vi "BIO_new.vi"(8 "error in (no error)":errorcluster, 10 "*BIO_method":u64, 11 "SSL-Lib in":refnum<class "SSL-Lib.lvclass">) -> (0 "error out":errorcluster, 2 "BIO out":refnum<class "BIO.lvclass">, 3 "SSL-Lib out":refnum<class "SSL-Lib.lvclass">)   [LabVIEW 2013, in "SSL_Lib.lvlib" / "SSL-Lib.lvclass"]
uses:
  SSL-Lib.lvclass
  BIO/BIO.lvclass
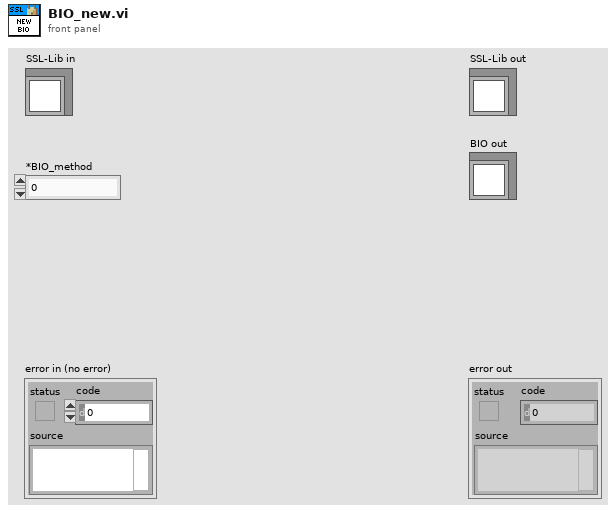
[diagram p1: front panel]
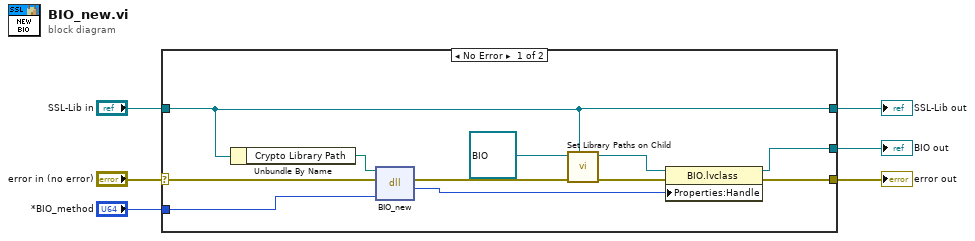
[diagram p0: block diagram]
diagram:
  n1 = case shown="No Error" "error in (no error)" {
    selector: "error in (no error)" -> [w17 w19]
    tunnel: [w10 w19] -> w5
    tunnel: [w12 w18] -> w3
    tunnel: "SSL-Lib in" -> [w12 w18]
    tunnel: "*BIO_method" -> [w15 _]
    tunnel: [w8 _] -> w1
    frame No Error {
      n2 = Unbundle By Name(w12) -> ("Crypto Library Path"=w16:path)
      n3 = dll-call lib="C:/Program Files (x86)/National Instruments/Shared/nissl/NIlibeay32.dll" fn="BIO_new"(path in=w16, error in=w17, "BIO_method"=w15) -> (error out=w13:errorcluster, "return type"=w7:u64)  [unwired: 2 in, 1 out]
      n4 = call-dynamic "Set Library Paths on Child.vi"(7:"SSL-Lib in"=w12, "error in (no error)"=w13, 11:"SSL-Lib in"=refnum<class "BIO.lvclass"> refnum ("SSL_Lib.lvlib:BIO.lvclass")) -> ("error out"=w11:errorcluster, "SSL-Lib out"=w9:refnum<class "BIO.lvclass">)  [unwired: 7 in]
      n5 = property class="BIO.lvclass"(reference=w9, error in=w11, "Properties:Handle"=w7) -> (reference out=w8:refnum<class "BIO.lvclass">, error out=w10:errorcluster)
    }
    frame Error {
    }
  }
  "error out" <- w5
  "SSL-Lib out" <- w3
  "BIO out" <- w1
